vi "Fichero.vi"() -> ()   [LabVIEW 2020]
uses:
  <vilib>/numeric/Random Number (Range) DBL.vi
panel:
  in  "String":string
  in  "Stop Button":bool
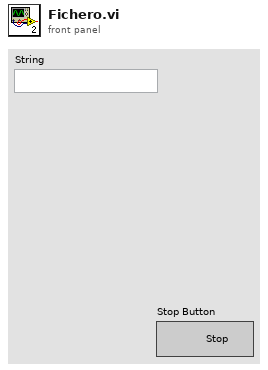
[diagram p1: front panel]
types:
  T1 = enum16{"open", "replace", "create", "open or create", "replace or create", "replace or create with confirmation"}
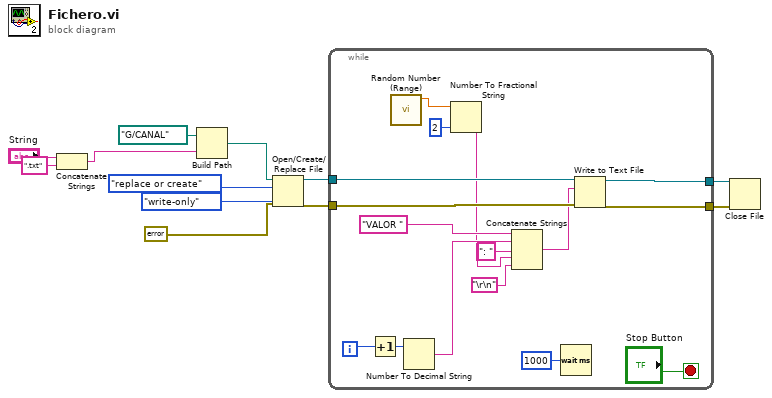
[diagram p0: block diagram]
diagram:
  n1 = Concatenate Strings("String", ".txt" ("string")) -> (w1:string)
  n2 = Build Path(base path=path "G:/CANAL", name or relative path=w1) -> (appended path=w7:path)
  n3 = Open/Create/Replace File(file path (use dialog)=w7, error in=errorcluster {"status"=FALSE, "code"=0, "source"=""} ("error constant"), operation (0:open)=T1."replace or create", access (0:read/write)=enum16{"read/write", "read-only", "write-only"}."write-only") -> (refnum out=w12:refnum<file>, error out=w11:errorcluster)  [unwired: 2 in, 1 out]
  n4 = while {
    tunnel: w12 -> [w26]
    tunnel: w11 -> [w25]
    tunnel: [w24] -> w10
    tunnel: [w23] -> w9
    i -> [w14]
    stop <- "Stop Button" stop-if-true
    n5 = Increment(x=w14) -> (x+1=w13:i32)
    n6 = call-poly <vilib>:"Random Number (Range).vi"() -> ("number"=w19:dbl)  [unwired: 11 in]
    n7 = Number To Decimal String(number=w13) -> (decimal integer string=w21:string)  [unwired: 1 in]
    n8 = Number To Fractional String(number=w19, precision (6)=i16 2) -> (F-format string=w17:string)  [unwired: 2 in]
    n9 = Concatenate Strings("VALOR ", w21, ": " ("string"), w17, "\r\n") -> (w15:string)
    n10 = Wait (ms)(milliseconds to wait=u32 1000) -> ()  [unwired: 1 out]
    n11 = Write to Text File(file (use dialog)=w26, text=w15, error in=w25) -> (refnum out=w24:refnum<file>, error out=w23:errorcluster)  [unwired: 1 in, 1 out]
  }
  n12 = Close File(refnum=w10, error in=w9) -> ()  [unwired: 2 out]
